vi "Global Variables.vi"() -> ()   [LabVIEW 2019]
panel:
  in  "Interpol. Dist. (µm)":dbl=0.1
  in  "Size":cluster{"Width":dbl, "Height":dbl}={"Width"=20.0, "Height"=20.0}
  in  "Offset":cluster{"Width":dbl, "Height":dbl}
  in  "Inkscape Ratio":dbl=1.0
  # "The default values of these have to have more elements than the number of paths you want.  This is dumb...."
  # "1"
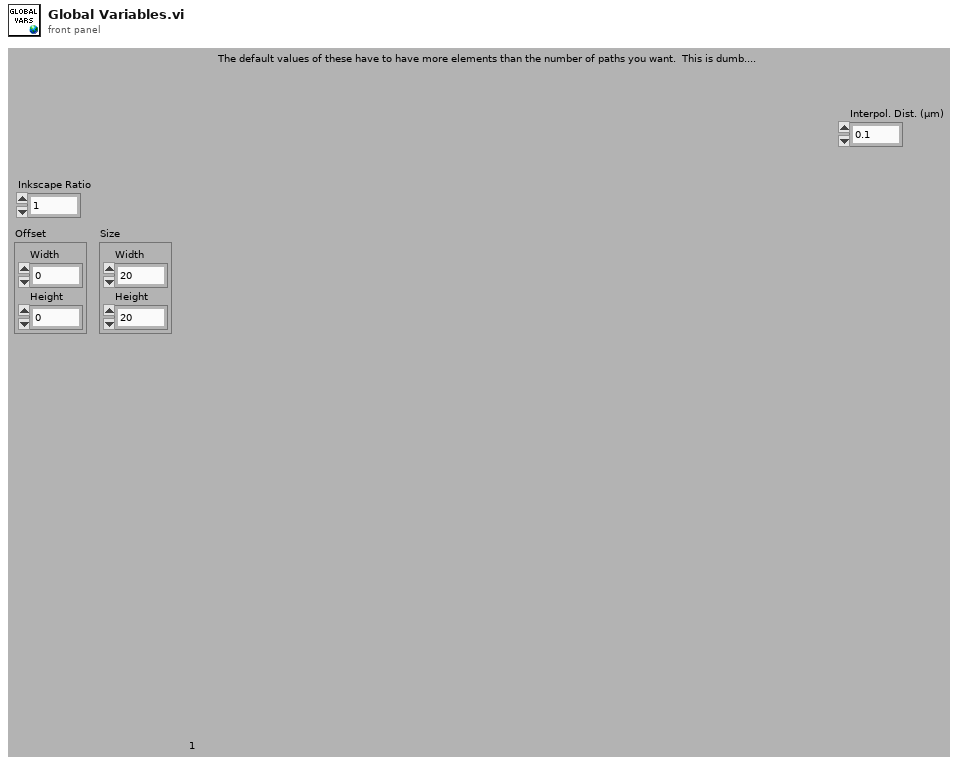
[diagram p1: front panel]
diagram:
